vi "Main.vi"(10 "Productos Subpanel":refnum<vi>, 11 "Module Admin":refnum<class "Delacor_lib_QMH_Module Admin.lvclass">) -> ()   [LabVIEW 2020, in "Productos.lvlib"]
doc: "This template is based off of the Queued Message Handler design pattern and the Queued Message Handler project template that ships with LabVIEW.\n\nThe main difference is that the queue is private to this module and communication between modules is performed via Broadcast and Request events.\n\nRequest events are wrapped in public API methods and are handled in the Event Handling Loop (EHL) of this VI. Any module can register for Broadcast events sent by this module. The EHL generates messages based on user interface actions.\n\nThe Message Handling Loop (MHL) processes messages generated by the EHL, or by other messages. The messages are string values, so new messages can be added easily to the Message Cases case structure in the MHL. Each message cluster can also provide an optional value for Message Data, which is a variant that can be converted to whatever message-specific data is required.\n_____\nBased on Delacor QMH Project Template 5.0.0.82."
uses:
  Productos.lvlib
  <vilib>/Delacor/Delacor QMH/Libraries/Module Admin_class/Delacor_lib_QMH_Module Admin.lvclass
  Module Data--cluster.ctl
  Stop Argument--cluster.ctl
  <vilib>/Delacor/Delacor QMH/Libraries/Message Queue_class/Delacor_lib_QMH_Message Queue.lvclass/Delacor_lib_QMH_Message Queue.ctl
  <vilib>/Delacor/Delacor QMH/Libraries/Module Admin_class/Delacor_lib_QMH_Module Admin.lvclass/Delacor_lib_QMH_Module Admin.ctl
  Set Products Argument--cluster.ctl
  Product Selection Argument--cluster.ctl
  <vilib>/Delacor/Delacor QMH/Libraries/Message Queue_class/Delacor_lib_QMH_Enqueue Message (Single).vi
  <vilib>/Delacor/Delacor QMH/Libraries/Module Admin_class/Delacor_lib_QMH_Get External Launch.vi
  <vilib>/Utility/error.llb/Error Cluster From Error Code.vi
  <vilib>/ErrorRing/Error Ring.xnode
  <vilib>/Delacor/Delacor QMH/Libraries/Message Queue_class/Delacor_lib_QMH_Message Queue.lvclass
  Coins/Coins.lvlib
  Messages/Messages.lvlib
panel:
  in  "Comprar":bool
  in  "Productos":i32(listbox)
  out "error out":errorcluster
  out "Status":string
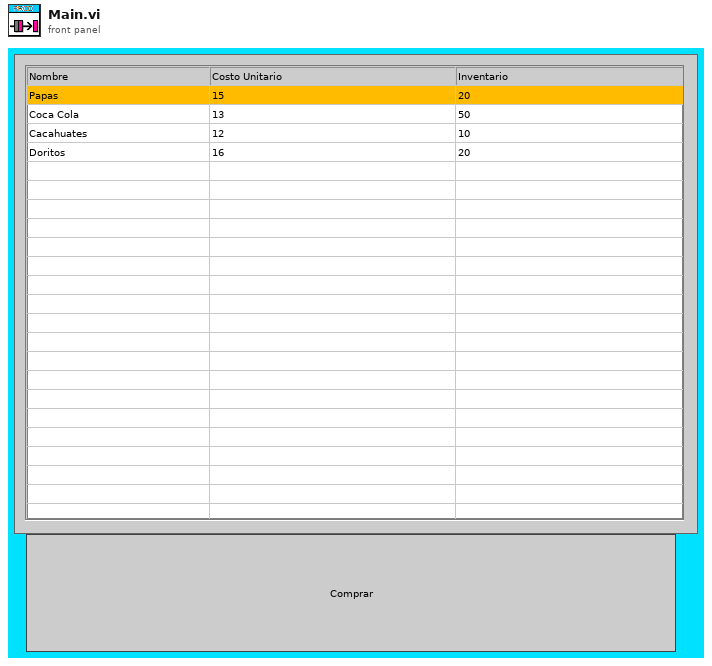
[diagram p1: front panel]
types:
  T1 = typedef "Productos.lvlib/Request Events--cluster.ctl" = cluster{"Stop Module":refnum<user-event>, "Show Panel":refnum<user-event>, "Hide Panel":refnum<user-event>, "Get Module Execution Status":refnum<user-event>, "Show Diagram":refnum<user-event>, "Set Products":refnum<user-event>, "Product Selection":refnum<user-event>}
  T2 = typedef "Coins.lvlib/Broadcast Events--cluster.ctl" = cluster{"Module Did Init":refnum<user-event>, "Status Updated":refnum<user-event>, "Error Reported":refnum<user-event>, "Module Did Stop":refnum<user-event>, "Update Module Execution Status":refnum<user-event>}
  T3 = typedef "Productos.lvlib/Module Data--cluster.ctl" = cluster{"Status":string, "Credito":dbl, "Nombre Productos":string[][], "Lista Ref":refnum<vi>, "Inventario":dbl, "Precio":dbl}
  T4 = enum32{"invalid lock state", "Not Locked", "Locked (No Password)", "Password-protected"}
  T5 = typedef "Productos.lvlib/Stop Argument--cluster.ctl" = cluster{"Origin":string, "Exit via Stop Module Req?":bool, "Wait for Module to stop?":bool}
  T6 = typedef "Productos.lvlib/Set Products Argument--cluster.ctl" = cluster{"Productos":string[][]}
  T7 = typedef "Productos.lvlib/Product Selection Argument--cluster.ctl" = cluster{"Numeric":i32}
  T8 = enum32{"Invalid", "Standard", "Closed", "Hidden", "Minimized", "Maximized"}
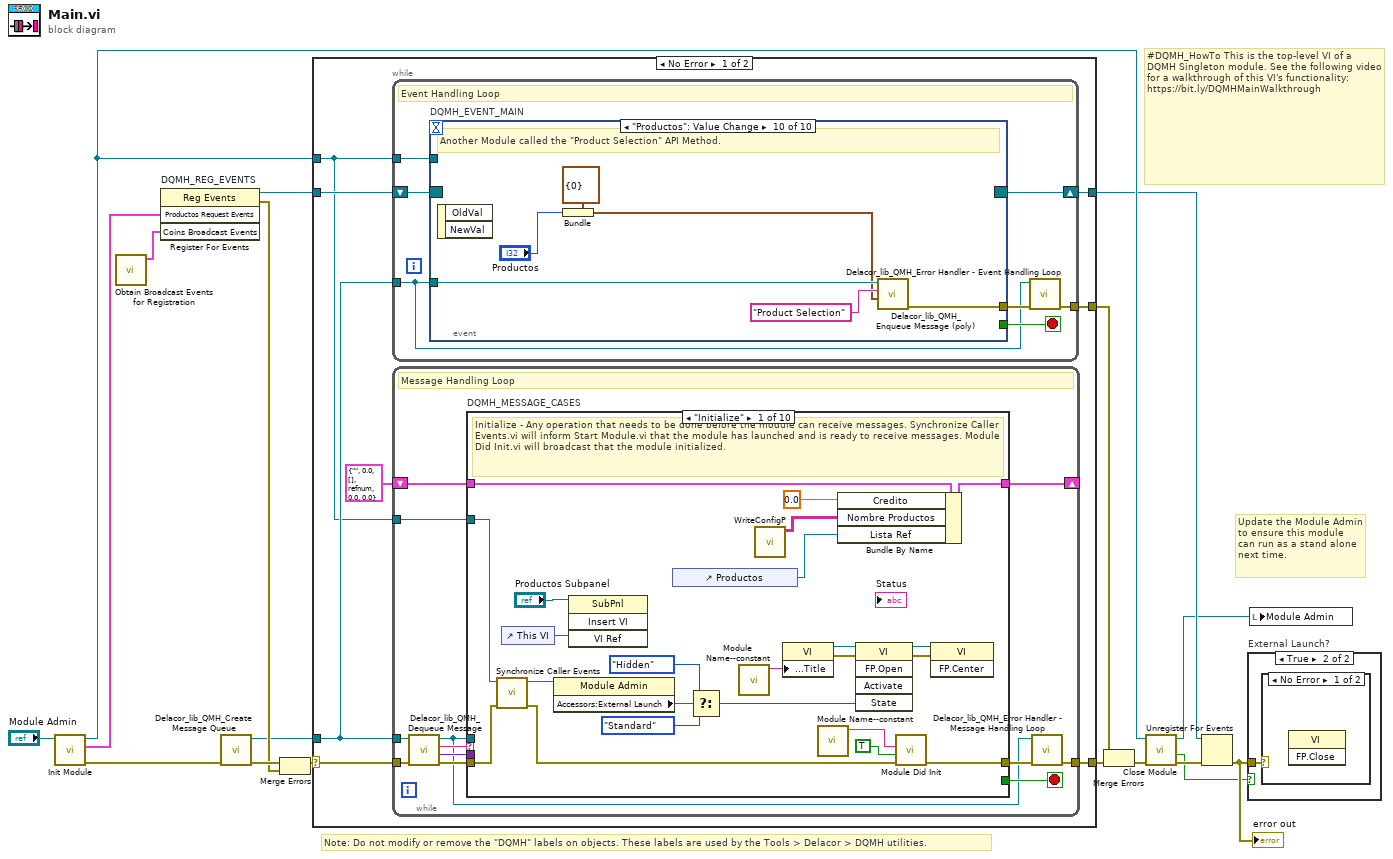
[diagram p0: block diagram]
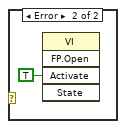
[diagram p3: hidden frame]
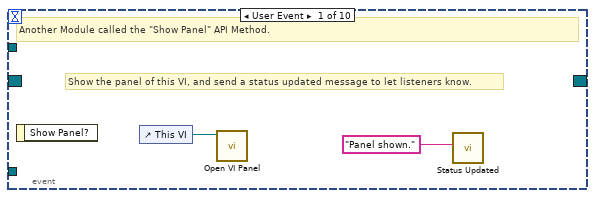
[diagram p4: hidden frame]
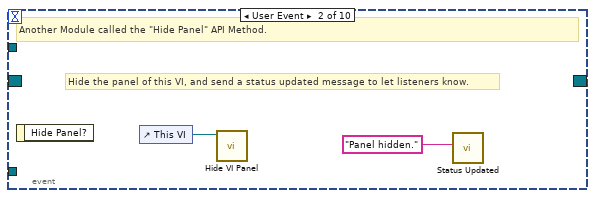
[diagram p5: hidden frame]
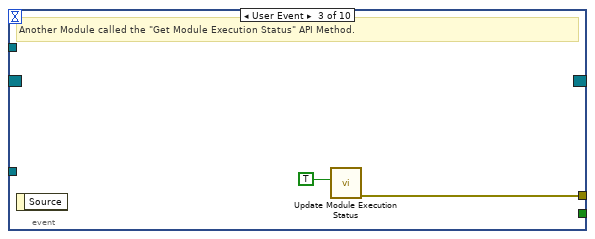
[diagram p6: hidden frame]
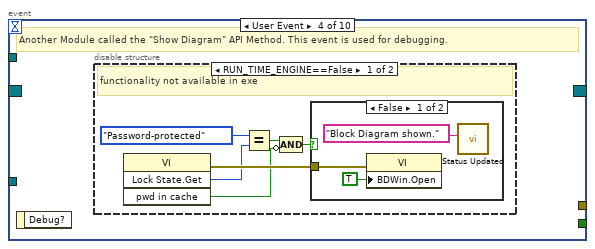
[diagram p7: hidden frame]
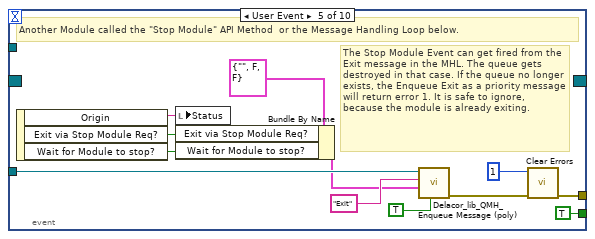
[diagram p10: hidden frame]
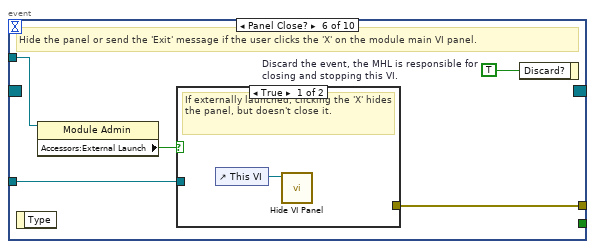
[diagram p11: hidden frame]
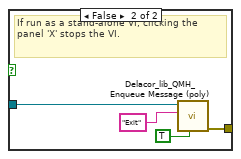
[diagram p12: hidden frame]
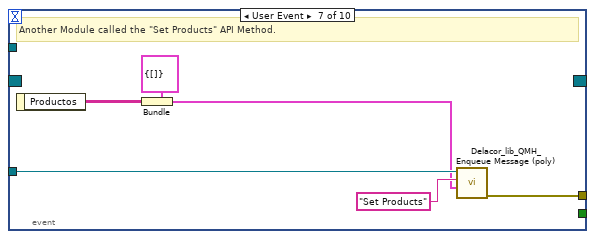
[diagram p13: hidden frame]
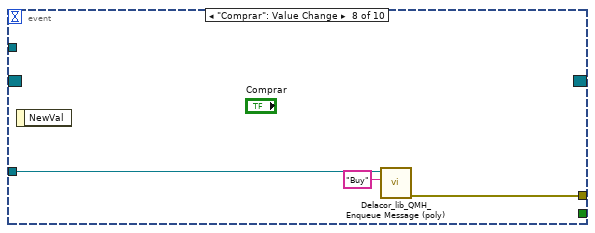
[diagram p14: hidden frame]
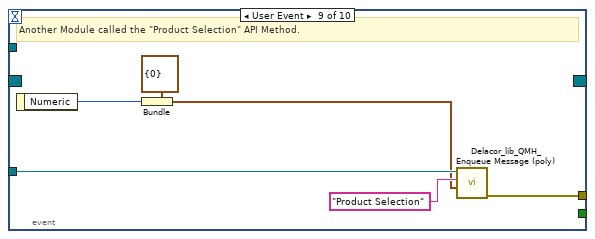
[diagram p15: hidden frame]
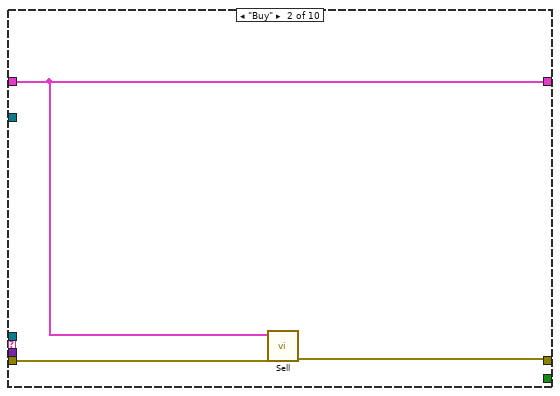
[diagram p16: hidden frame]
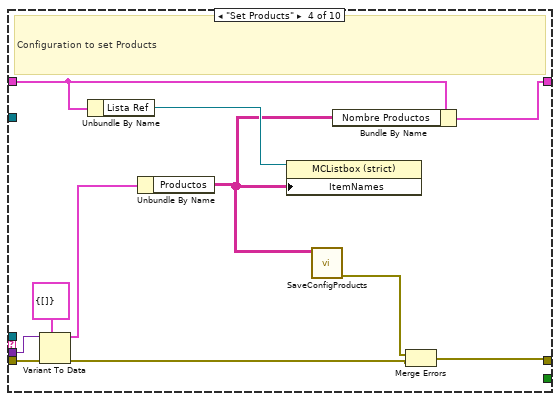
[diagram p18: hidden frame]
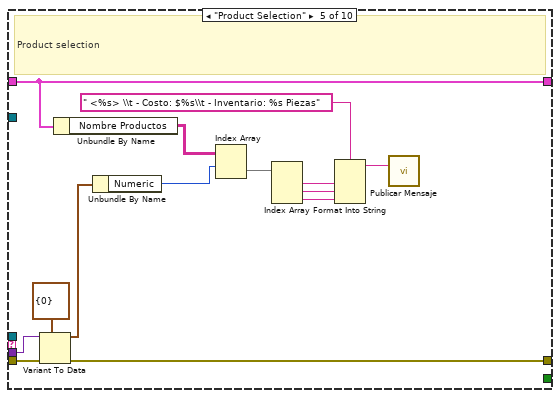
[diagram p19: hidden frame]
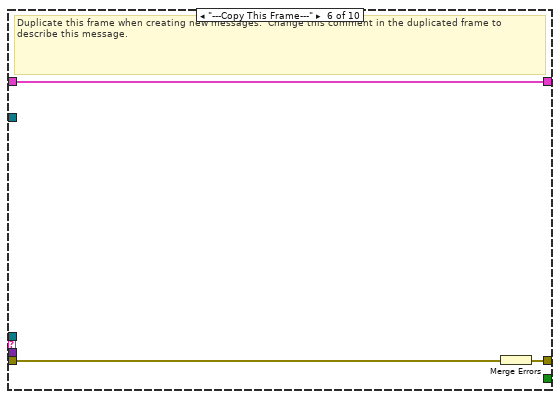
[diagram p20: hidden frame]
diagram:
  # "#DQMH_HowTo This is the top-level VI of a DQMH Singleton module. See the following video for a walkthrough of this VI's functionality: https://bit.ly/DQMHMainWalkthrough"
  # "Note: Do not modify or remove the \"DQMH\" labels on objects. These labels are used by the Tools > Delacor > DQMH utilities."
  # "Update the Module Admin to ensure this module can run as a stand alone next time."
  n1 = call "Init Module.vi"("Singleton Module Admin in"="Module Admin") -> ("error out"=w17:errorcluster, "Productos Request Events"=w6:T1, "Singleton Module Admin out"=w9:refnum<class "Delacor_lib_QMH_Module Admin.lvclass">)  [unwired: 8 in]
  n2 = call "Obtain Broadcast Events for Registration.vi"() -> ("Coins Broadcast Events"=w1:T2)  [unwired: 9 in, 2 out]
  n3 = register-events "DQMH_REG_EVENTS"(w6, w1) -> (reference out=w7:refnum<event-registration>, error out=w10:errorcluster)  [unwired: 2 in]
  n4 = call <vilib>:"Delacor_lib_QMH_Create Message Queue.vi"("error in (no error)"=w17) -> ("error out"=w12:errorcluster, "Message Queue"=w5:refnum<class "Delacor_lib_QMH_Message Queue.lvclass">)  [unwired: 9 in]
  n5 = Merge Errors(w12, w10) -> (w11:errorcluster)
  n6 = case shown="No Error" w11 {
    selector: w11 -> [w24 w210]
    tunnel: [w26 w209] -> w18
    tunnel: [w23 w215] -> w8
    tunnel: w7 -> [w21 w215]
    tunnel: w5 -> [w20 w208]
    tunnel: [w25 _] -> w15
    tunnel: w9 -> [w19 w211]
    frame No Error {
      n7 = while {
        tunnel: w20 -> [w27]
        shift-right: [w30] -> w23
        shift-left: w21 -> [w31]
        tunnel: [w32] -> w25
        tunnel: w19 -> [w28]
        stop <- w29 stop-if-true
        # "Event Handling Loop"
        n8 = event "DQMH_EVENT_MAIN" shown="[9] \"Productos\": Value Change" {
          selector: w31 -> [_ _ _ _ _ _ _ _ _ _]
          dyn-events: [_ _ _ _ _ _ _ _ _ _] -> w30
          timeout: _ -> [_ _ _ _ _ _ _ _ _ _]
          tunnel: [_ _ _ _ TRUE ("Discard?") _ _ _ _ _] -> w29
          tunnel: w27 -> [_ _ _ _ w56 w63 w76 w79 w85 w91]
          tunnel: [_ _ w39 _ w59 w65 w71 w78 w80 w88] -> w33
          tunnel: w28 -> [_ _ _ _ _ w62 _ _ _ _]
          event User Event {
            # "Show the panel of this VI, and send a status updated message to let listeners know."
            # "Another Module called the \"Show Panel\" API Method."
            n9 = event-data() -> ()  [unwired: 1 in, 1 out]
            n10 = control-ref of="This VI"() -> (w35:refnum<vi>)
            n11 = call "Open VI Panel.vi"("VI"=w35) -> ()  [unwired: 10 in, 1 out]
            n12 = call "Status Updated.vi"("Status"="Panel shown." ("format string")) -> ()  [unwired: 10 in, 1 out]
          }
          event User Event {
            # "Hide the panel of this VI, and send a status updated message to let listeners know."
            # "Another Module called the \"Hide Panel\" API Method."
            n13 = event-data() -> ()  [unwired: 1 in, 1 out]
            n14 = control-ref of="This VI"() -> (w37:refnum<vi>)
            n15 = call "Hide VI Panel.vi"("VI"=w37) -> ()  [unwired: 10 in, 1 out]
            n16 = call "Status Updated.vi"("Status"="Panel hidden." ("format string")) -> ()  [unwired: 10 in, 1 out]
          }
          event User Event {
            # "Another Module called the \"Get Module Execution Status\" API Method."
            n17 = event-data() -> ()  [unwired: 1 in, 1 out]
            n18 = call "Update Module Execution Status.vi"("Running?"=TRUE) -> ("error out"=w39:errorcluster)  [unwired: 10 in]
          }
          event User Event {
            # "Another Module called the \"Show Diagram\" API Method. This event is used for debugging."
            n19 = event-data() -> ()  [unwired: 1 in, 1 out]
            n20 = disable-structure shown="RUN_TIME_ENGINE==False" {
              frame condition #0 (active) {
                # "functionality not available in exe"
                n21 = invoke class="VI" method="Lock State.Get"() -> (error out=w45:errorcluster, "Get Lock State"=w44:T4, "pwd in cache"=w41:bool)  [unwired: 4 in, 1 out]
                n22 = Equal?(x=T4."Password-protected", y=w44) -> (x = y?=w42:bool)
                n23 = Compound Arithmetic op=AND(w42, invert w41) -> (w40:bool)
                n24 = case shown="False" w40 {
                  tunnel: w45 -> [w48 _]
                  frame False {
                    n25 = property class="VI"(error in=w48, "BDWin.Open"=TRUE ("Block Diagram Window:Open")) -> ()  [unwired: 1 in, 2 out]
                    n26 = call "Status Updated.vi"("Status"="Block Diagram shown." ("format string")) -> ()  [unwired: 10 in, 1 out]
                  }
                  frame True {
                    # "Password-protected VI, and the password is not in the cache. Do not show the diagram."
                  }
                }
              }
              frame condition #1 {
              }
            }
          }
          event User Event {
            # "The Stop Module Event can get fired from the Exit message in the MHL. The queue gets destroyed in that case. If the queue no longer exists, the Enqueue Exit as a priority message will return error 1. It is safe to ignore, because the module is already exiting."
            # "Another Module called the \"Stop Module\" API Method  or the Message Handling Loop below."
            n27 = event-data() -> ("Origin"=w55:string, "Exit via Stop Module Req?"=w51:bool, "Wait for Module to stop?"=w50:bool)  [unwired: 1 in]
            n28 = local write "Status"(w55) -> ()
            n29 = Bundle By Name(cluster=T5 {"Origin"="", "Exit via Stop Module Req?"=FALSE, "Wait for Module to stop?"=FALSE} ("Stop Argument"), "Exit via Stop Module Req?"=w51, "Wait for Module to stop?"=w50) -> (w49:T5)
            n30 = call-poly <vilib>:"Delacor_lib_QMH_Enqueue Message (poly).vi"("Priority Message? (F)"=TRUE, "Message Data"=w49, "Message"="Exit", "Message Queue in"=w56) -> ("error out"=w60:errorcluster)  [unwired: 6 in, 1 out]
            n31 = call <vilib>:"Clear Errors.vi"("error in (no error)"=w60, "specific error code to clear (0: all)"=1) -> ("error out"=w59:errorcluster)  [unwired: 4 in, 1 out]
          }
          event Panel Close? {
            w64 = TRUE  # Discard the event, the MHL is responsible for closing and stopping this VI.
            # "Hide the panel or send the 'Exit' message if the user clicks the 'X' on the module main VI panel."
            n32 = event-data() -> ()  [unwired: 1 in, 1 out]
            n33 = property class="Module Admin"(reference=w62) -> ("Accessors:External Launch"=w61:bool)  [unwired: 1 in, 2 out]
            n34 = case shown="True" w61 {
              tunnel: w63 -> [_ w69]
              tunnel: [_ w70] -> w65
              frame True {
                # "If externally launched, clicking the 'X' hides the panel, but doesn't close it."
                n35 = control-ref of="This VI"() -> (w66:refnum<vi>)
                n36 = call "Hide VI Panel.vi"("VI"=w66) -> ()  [unwired: 10 in, 1 out]
              }
              frame False {
                # "If run as a stand-alone VI, clicking the panel 'X' stops the VI."
                n37 = call-poly <vilib>:"Delacor_lib_QMH_Enqueue Message (poly).vi"("Priority Message? (F)"=TRUE, "Message"="Exit", "Message Queue in"=w69) -> ("error out"=w70:errorcluster)  [unwired: 7 in, 1 out]
              }
            }
            n38 = event-data("Discard?"=w64) -> ()  [unwired: 1 in, 1 out]
          }
          event User Event {
            # "Another Module called the \"Set Products\" API Method."
            n39 = event-data() -> ("Productos"=w72:string[][])  [unwired: 1 in]
            n40 = Bundle(cluster=T6 {"Productos"=[]} ("Set Products Argument"), "Productos"=w72) -> (w73:T6)
            n41 = call-poly <vilib>:"Delacor_lib_QMH_Enqueue Message (poly).vi"("Message Data"=w73, "Message"="Set Products", "Message Queue in"=w76) -> ("error out"=w71:errorcluster)  [unwired: 7 in, 1 out]
          }
          event "Comprar": Value Change {
            n42 = event-data() -> ()  [unwired: 1 in, 1 out]
            n43 = call-poly <vilib>:"Delacor_lib_QMH_Enqueue Message (poly).vi"("Message"="Buy", "Message Queue in"=w79) -> ("error out"=w78:errorcluster)  [unwired: 8 in, 1 out]
          }
          event User Event {
            # "Another Module called the \"Product Selection\" API Method."
            n44 = event-data() -> ("Numeric"=w81:i32)  [unwired: 1 in]
            n45 = Bundle(cluster=T7 {"Numeric"=0} ("Product Selection Argument"), "Numeric"=w81) -> (w82:T7)
            n46 = call-poly <vilib>:"Delacor_lib_QMH_Enqueue Message (poly).vi"("Message Data"=w82, "Message"="Product Selection", "Message Queue in"=w85) -> ("error out"=w80:errorcluster)  [unwired: 7 in, 1 out]
          }
          event "Productos": Value Change {
            # "Another Module called the \"Product Selection\" API Method."
            n47 = event-data() -> ()  [unwired: 1 in, 2 out]
            n48 = Bundle(cluster=T7 {"Numeric"=0} ("Product Selection Argument"), "Numeric"="Productos") -> (w86:T7)
            n49 = call-poly <vilib>:"Delacor_lib_QMH_Enqueue Message (poly).vi"("Message Data"=w86, "Message"="Product Selection", "Message Queue in"=w91) -> ("error out"=w88:errorcluster)  [unwired: 7 in, 1 out]
          }
        }
        n50 = call-dynamic "Delacor_lib_QMH_Error Handler - Event Handling Loop.vi"("error in (no error)"=w33, "Message Queue in"=w27) -> ("dup error in"=w32:errorcluster)  [unwired: 8 in, 1 out]
      }
      n51 = while {
        tunnel: w20 -> [w94]
        shift-right: [w98] -> _
        shift-left: T3 {"Status"="", "Credito"=0.0, "Nombre Productos"=[], "Lista Ref"=refnum, "Inventario"=0.0, "Precio"=0.0} ("Data Cluster") -> [w99]
        tunnel: w24 -> [w102]
        tunnel: [w100] -> w26
        tunnel: w19 -> [w92]
        stop <- w97 stop-if-true
        # "Message Handling Loop"
        n52 = call-dynamic "Delacor_lib_QMH_Dequeue Message.vi"("error in (no error)"=w102, "Message Queue in"=w94) -> ("error out"=w101:errorcluster, "Message Data"=w95:variant, "Message"=w96:string, "Message Queue out"=w93:refnum<class "Delacor_lib_QMH_Message Queue.lvclass">)  [unwired: 6 in]
        n53 = case "DQMH_MESSAGE_CASES" shown="\"Initialize\"" w96 {
          selector: w96 -> [_ _ _ _ _ _ _ _ _ w195]
          tunnel: w93 -> [_ _ _ _ _ _ _ w165 w187 _]
          tunnel: w101 -> [w124 w129 w131 w142 w156 w159 w161 w172 w193 w197]
          tunnel: [w122 w128 w131 w133 w155 w158 w161 w168 w190 w198] -> w103
          tunnel: w99 -> [w113 w127 w130 w137 w151 w157 w160 w167 w186 w196]
          tunnel: [w112 w127 w130 w136 w151 w157 w160 w167 w186 w196] -> w98
          tunnel: [_ _ _ _ _ _ _ _ w185 _] -> w97
          tunnel: w95 -> [_ _ _ w141 w154 _ _ w166 w184 _]
          tunnel: w92 -> [w114 _ _ _ _ _ _ w164 w179 _]
          frame "Initialize" {
            # "Initialize - Any operation that needs to be done before the module can receive messages. Synchronize Caller Events.vi will inform Start Module.vi that the module has launched and is ready to receive messages. Module Did Init.vi will broadcast that the module initialized."
            n54 = call "Synchronize Caller Events.vi"("error in (no error)"=w124, "Singleton Module Admin in"=w114) -> ("error out"=w123:errorcluster, "Singleton Module Admin out"=w109:refnum<class "Delacor_lib_QMH_Module Admin.lvclass">)  [unwired: 8 in]
            n55 = control-ref of="This VI"() -> (w107:refnum<vi>)
            n56 = property class="Module Admin"(reference=w109) -> ("Accessors:External Launch"=w118:bool)  [unwired: 1 in, 2 out]
            n57 = invoke class="SubPnl" method="Insert VI"(reference="Productos Subpanel", "VI Ref"=w107) -> ()  [unwired: 2 in, 4 out]
            n58 = control-ref of="Productos"() -> (w104:refnum<vi>)
            n59 = Select(t=T8."Hidden" ("State"), s=w118, f=T8."Standard" ("State")) -> (s? t:f=w115:T8)
            n60 = call "Module Name--constant.vi"() -> ("Module Name"=w121:string)  [unwired: 11 in]
            n61 = call "WriteConfigP.vi"() -> ("Array"=w105:string[][])  [unwired: 10 in, 1 out]
            n62 = property class="VI"("Front Panel.Title"=w121) -> (reference out=w120:refnum<vi>, error out=w126:errorcluster)  [unwired: 2 in]
            n63 = call "Module Name--constant.vi"() -> ("Module Name"=w110:string)  [unwired: 11 in]
            n64 = Bundle By Name(cluster=w113, "Credito"=0.0, "Nombre Productos"=w105, "Lista Ref"=w104) -> (w112:T3)
            n65 = invoke class="VI" method="FP.Open"(reference=w120, error in=w126, "State"=w115) -> (reference out=w119:refnum<vi>, error out=w125:errorcluster)  [unwired: 2 in, 3 out]
            n66 = call "Module Did Init.vi"("error in (no error)"=w123, "Initialized?"=TRUE, "Origin"=w110) -> ("error out"=w122:errorcluster)  [unwired: 8 in]
            n67 = invoke class="VI" method="FP.Center"(reference=w119, error in=w125) -> ()  [unwired: 1 in, 3 out]
          }
          frame "Buy" {
            n68 = call "Sell.vi"("error in (no error)"=w129, "Data cluster"=w127) -> ("error out"=w128:errorcluster)  [unwired: 9 in]
          }
          frame "--- Module Specific ---" {
            # "Separator -- The following cases handle messages specific to this Module."
          }
          frame "Set Products" {
            # "Configuration to set Products"
            n69 = Variant To Data(error in=w142, type=T6 {"Productos"=[]} ("Set Products Argument"), Variant=w141) -> (data=w139:T6, error out=w134:errorcluster)
            n70 = Unbundle By Name(w137) -> ("Lista Ref"=w138:refnum<vi>)
            n71 = Unbundle By Name(w139) -> ("Productos"=w135:string[][])
            n72 = property class="MCListbox (strict)"(reference=w138, "ItemNames"=w135) -> ()  [unwired: 1 in, 2 out]
            n73 = call "SaveConfigProducts.vi"("Products"=w135) -> ("error out"=w132:errorcluster)  [unwired: 10 in]
            n74 = Bundle By Name(cluster=w137, "Nombre Productos"=w135) -> (w136:T3)
            n75 = Merge Errors(w132, w134) -> (w133:errorcluster)
          }
          frame "Product Selection" {
            # "Product selection"
            n76 = Variant To Data(error in=w156, type=T7 {"Numeric"=0} ("Product Selection Argument"), Variant=w154) -> (data=w152:T7, error out=w155:errorcluster)
            n77 = Unbundle By Name(w151) -> ("Nombre Productos"=w150:string[][])
            n78 = Unbundle By Name(w152) -> ("Numeric"=w149:i32)
            n79 = Index Array(array=w150, index (row)=w149) -> (element=w148:string[])  [unwired: 1 in]
            n80 = Index Array(array=w148) -> (element #1=w147:string, element #2=w146:string, element #3=w145:string)  [unwired: 3 in]
            n81 = Format Into String(format string=" <%s> \\t - Costo: $%s\\t - Inventario: %s Piezas", w147, w146, w145) -> (resulting string=w144:string)  [unwired: 2 in, 1 out]
            n82 = call "Publicar Mensaje.vi"("Mensaje"=w144) -> ()  [unwired: 10 in, 1 out]
          }
          frame "---Copy This Frame---" {
            # "Duplicate this frame when creating new messages.  Change this comment in the duplicated frame to describe this message."
            n83 = Merge Errors(w159) -> (w158:errorcluster)
          }
          frame "--- Exit and Error Handling---" {
            # "Separator - The following cases handle errors and exit messages."
          }
          frame "Error" {
            # "#CodeRecommended - If you ever change the name of this \"Error\" message, you'll need to update the name in the Check Loop Error.vi as well."
            # "#CodeRecommended - If the module is running in standalone mode (External Launch = FALSE), this code will pop up an error dialog and call the 'Exit' message if an error occurs. Add more fine-grained error handling here."
            # "Error - Check the error message data and respond accordingly. This message is sent by the \"Error Handler\" VIs at the end of each loop in this application."
            n84 = property class="Module Admin"(reference=w164) -> ("Accessors:External Launch"=w163:bool)  [unwired: 1 in, 2 out]
            n85 = Variant To Data(error in=w172, type=errorcluster {"status"=FALSE, "code"=0, "source"=""} ("error constant"), Variant=w166) -> (data=w173:errorcluster, error out=w170:errorcluster)
            n86 = call "Module Name--constant.vi"() -> ("Module Name"=w162:string)  [unwired: 11 in]
            n87 = call "Error Reported.vi"("Additional Information"=w162, "Error"=w173) -> ()  [unwired: 9 in, 1 out]
            n88 = case shown="False" w163 {
              tunnel: [w178 _] -> w169
              tunnel: w165 -> [w176 _]
              tunnel: w173 -> [w177 _]
              frame False {
                # "If the module is running standalone, then pop up an error dialog and call the \"Exit\" message."
                n89 = call <vilib>:"Simple Error Handler.vi"("error in (no error)"=w177) -> ()  [unwired: 4 in, 5 out]
                n90 = call-poly <vilib>:"Delacor_lib_QMH_Enqueue Message (poly).vi"("Priority Message? (F)"=TRUE, "Message"="Exit", "Message Queue in"=w176) -> ("error out"=w178:errorcluster)  [unwired: 7 in, 1 out]
              }
              frame True {
                # "If the module was launched externally, calling the Error Reported broadcast VI is the only action performed by the \"Error\" message. The module's caller can then process the error appropriately."
              }
            }
            n91 = Merge Errors(w170, w169) -> (w168:errorcluster)
            n92 = local write "error out"(w168) -> ()
          }
          frame "Exit" {
            w183 = 91  # 91: not all Exit messages will have an argument
            w185 = TRUE  # Stop the VI
            # "Release the message queue reference"
            # "#CodeNeeded - Add any required cleanup code here"
            # "Exit - Exit the application."
            n93 = Variant To Data(error in=w193, type=T5 {"Origin"="", "Exit via Stop Module Req?"=FALSE, "Wait for Module to stop?"=FALSE} ("Stop Argument"), Variant=w184) -> (data=w181:T5, error out=w189:errorcluster)
            n94 = call <vilib>:"Clear Errors.vi"("error in (no error)"=w189, "specific error code to clear (0: all)"=w183) -> ("error out"=w192:errorcluster)  [unwired: 4 in, 1 out]
            n95 = control-ref of="This VI"() -> (w180:refnum<vi>)
            n96 = call-dynamic "Delacor_lib_QMH_Release Message Queue.vi"("error in (no error)"=w192, "Message Queue"=w187) -> ("error out"=w191:errorcluster)  [unwired: 9 in]
            n97 = call "Handle Exit.vi"("Stop Argument"=w181, "Admin in"=w179, "VI reference"=w180) -> ("error out"=w188:errorcluster)  [unwired: 7 in, 1 out]
            n98 = Merge Errors(w191, w188) -> (w190:errorcluster)
          }
          frame Default {
            # "'Default' case only runs if there is a message that isn't defined in any of the other cases.  Output a programming error."
            n99 = call "Module Name--constant.vi"() -> ("Module Name"=w194:string)  [unwired: 11 in]
            n100 = xnode "Error Ring"("parameter 0"=w195, "parameter 1"=w194) -> ("error out"=w199:errorcluster)
            n101 = Merge Errors(w197, w199) -> (w198:errorcluster)
          }
        }
        n102 = call-dynamic "Delacor_lib_QMH_Error Handler - Message Handling Loop.vi"("error in (no error)"=w103, "Message Queue in"=w93) -> ("dup error in"=w100:errorcluster)  [unwired: 8 in, 1 out]
      }
    }
    frame Error {
      # "Synchronize Caller Events.vi will inform Start Module.vi that the module has launched and will let the code calling Start Module.vi register for broadcasts and would permit the caller receive the broadcast that an error occurred at launch time."
      n103 = call-dynamic "Delacor_lib_QMH_Release Message Queue.vi"("error in (no error)"=w210, "Message Queue"=w208) -> ("error out"=w209:errorcluster)  [unwired: 9 in]
      n104 = call "Synchronize Caller Events.vi"("Singleton Module Admin in"=w211) -> ("error out"=w216:errorcluster)  [unwired: 9 in, 1 out]
      n105 = call "Module Name--constant.vi"() -> ("Module Name"=w214:string)  [unwired: 11 in]
      n106 = Format Into String(format string="An error occurred during initialization. %s is no longer running.", w214) -> (resulting string=w212:string)  [unwired: 2 in, 1 out]
      n107 = Merge Errors(w209, w216) -> (w217:errorcluster)
      n108 = call "Error Reported.vi"("Additional Information"=w212, "Error"=w217) -> ()  [unwired: 9 in, 1 out]
    }
  }
  n109 = Merge Errors(w15, w18) -> (w14:errorcluster)
  n110 = call "Close Module.vi"("error in (no error)"=w14, "Module Admin in"=w9) -> ("error out"=w16:errorcluster, "External Launch"=w2:bool, "Module Admin out"=w3:refnum<class "Delacor_lib_QMH_Module Admin.lvclass">)  [unwired: 7 in]
  n111 = Unregister For Events(event registration refnum=w8, error in=w16) -> (error out=w13:errorcluster)
  "error out" <- w13
  n112 = case "External Launch?" shown="True" w2 {
    tunnel: w13 -> [_ w218]
    frame False {
    }
    frame True {
      n113 = case shown="No Error" w218 {
        frame No Error {
          n114 = invoke class="VI" method="FP.Close"() -> ()  [unwired: 3 in, 3 out]
        }
        frame Error {
          n115 = invoke class="VI" method="FP.Open"("Activate"=TRUE ("Activate?")) -> ()  [unwired: 4 in, 5 out]
        }
      }
    }
  }
  n116 = local write "Module Admin"(w3) -> ()
